vi "Read session data.vi"(8 "error in (no error)":errorcluster, 11 "LIA Host Interface FPGA in":refnum<class "LIA Host Interface FPGA.lvclass">) -> (0 "error out":errorcluster, 2 "session data":refnum<data-value>, 3 "LIA Host Interface FPGA out":refnum<class "LIA Host Interface FPGA.lvclass">)   [LabVIEW 2017, in "LIA Host Interface FPGA.lvclass"]
uses:
  LIA Host Interface FPGA.lvclass
  Private/session data.ctl
  LIA Host Interface FPGA.lvclass/LIA Host Interface FPGA.ctl
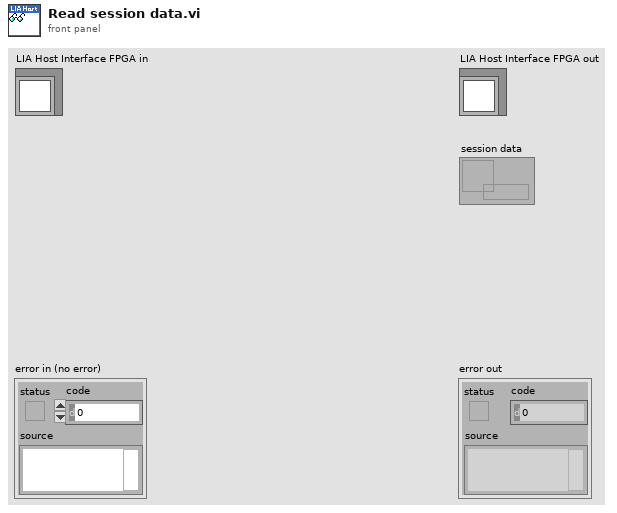
[diagram p1: front panel]
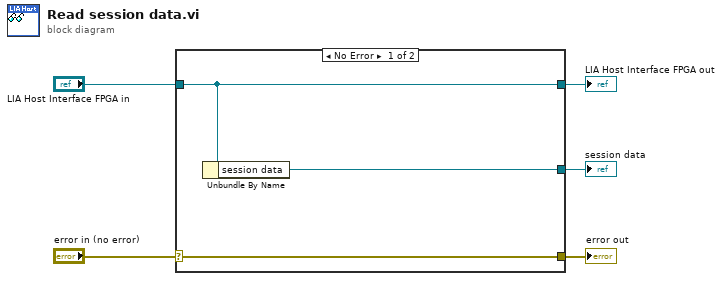
[diagram p0: block diagram]
diagram:
  n1 = case shown="No Error" "error in (no error)" {
    selector: "error in (no error)" -> [w8 w9]
    tunnel: [w8 w9] -> w4
    tunnel: [w7 w10] -> w2
    tunnel: "LIA Host Interface FPGA in" -> [w7 w10]
    tunnel: [w6 _] -> w1
    frame No Error {
      n2 = Unbundle By Name(w7) -> ("session data"=w6:refnum<data-value>)
    }
    frame Error {
    }
  }
  "error out" <- w4
  "LIA Host Interface FPGA out" <- w2
  "session data" <- w1
